vi "Do.vi"(8 "error in (no error)":errorcluster, 10 "Actor in":refnum<class "Actor.lvclass">, 11 "Configure Tranducer Type [TMP] Msg":refnum<class "Configure Tranducer Type [TMP] Msg.lvclass">) -> (0 "error out":errorcluster, 2 "Actor out":refnum<class "Actor.lvclass">)   [LabVIEW 2013, in "CS++DMM.lvlib" / "Configure Tranducer Type [TMP] Msg.lvclass"]
doc: "This VI delivers the message to the actor by calling the appropriate method(s) on the actor."
uses:
  Configure Tranducer Type [TMP] Msg.lvclass
  <vilib>/ActorFramework/Actor/Actor.lvclass
  CS++DMM/CS++DMM.lvclass
  Configure Tranducer Type [TMP] Msg.lvclass/Configure Tranducer Type [TMP] Msg.ctl
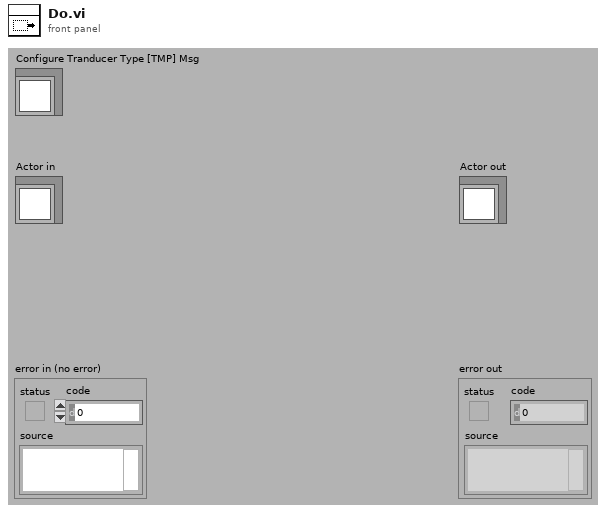
[diagram p1: front panel]
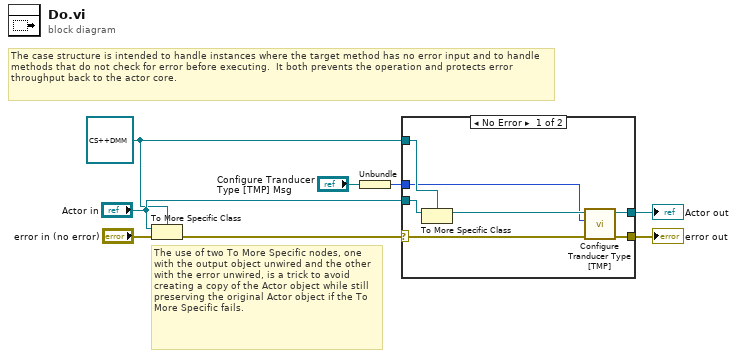
[diagram p0: block diagram]
diagram:
  w2 = refnum<class "CS++DMM.lvclass"> refnum ("Actor in")
  # "The use of two To More Specific nodes, one with the output object unwired and the other with the error unwired, is a trick to avoid creating a copy of the Actor object while still preserving the original Actor object if the To More Specific fails."
  # "The case structure is intended to handle instances where the target method has no error input and to handle methods that do not check for error before executing.  It both prevents the operation and protects error throughput back to the actor core."
  n1 = To More Specific Class(target class=w2, reference="Actor in", error in="error in (no error)") -> (error out=w6:errorcluster)  [unwired: 1 out]
  n2 = Unbundle("Configure Tranducer Type [TMP] Msg") -> (w1:i32)
  n3 = case shown="No Error" w6 {
    selector: w6 -> [w13 w17]
    tunnel: [w15 w17] -> w5
    tunnel: [w14 w16] -> w4
    tunnel: "Actor in" -> [w12 w16]
    tunnel: w2 -> [w11 _]
    tunnel: w1 -> [w9 _]
    frame No Error {
      n4 = To More Specific Class(target class=w11, reference=w12) -> (specific class reference=w10:refnum<class "CS++DMM.lvclass">)  [unwired: 1 in, 1 out]
      n5 = call "Configure Tranducer Type [TMP].vi"("error in (no error)"=w13, "transducer type (Thermocouple)"=w9, "CS++DMM in"=w10) -> ("error out"=w15:errorcluster, "CS++DMM out"=w14:refnum<class "CS++DMM.lvclass">)  [unwired: 7 in]
    }
    frame Error {
      # "If type check fails, pass the original object out again."
    }
  }
  "error out" <- w5
  "Actor out" <- w4
